vi "Change Speed.vi"(8 "error in (no error)":errorcluster, 10 "Mixer":i16(knob) scale=0.0..100.0, 11 "Feeder Actor.lvlib:Mixer.lvclass":refnum<class "Mixer.lvclass">) -> (0 "error out":errorcluster, 3 "Actor out":refnum<class "Actor.lvclass">)   [LabVIEW 2018, in "Feeder Actor.lvlib" / "Mixer.lvclass"]
uses:
  Mixer.lvclass
  C:/Program Files/National Instruments/LabVIEW 2018/vi.lib/ActorFramework/Actor/Actor.lvclass
  <vilib>/ActorFramework/Actor/Actor.lvclass
  Mixer.lvclass/Mixer.ctl
  <vilib>/DAQmx/write.llb/DAQmx Write (Counter Frequency 1Chan 1Samp).vi
  <vilib>/DAQmx/miscellaneous.llb/DAQmx Fill In Error Info.vi
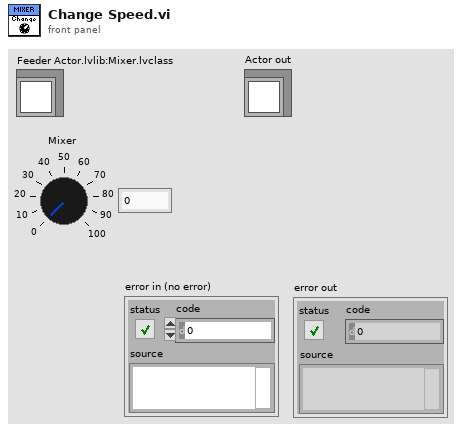
[diagram p1: front panel]
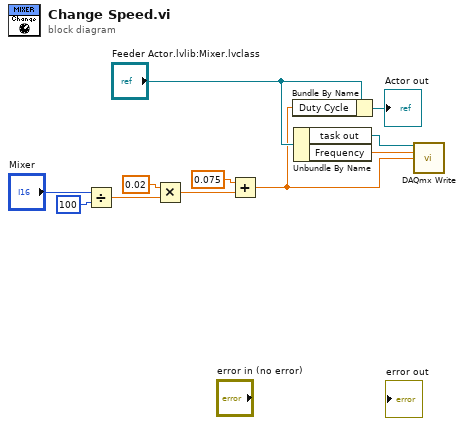
[diagram p0: block diagram]
diagram:
  n1 = Divide(x="Mixer", y=i16 100) -> (x/y=w7:dbl)
  n2 = Multiply(x=0.02, y=w7) -> (x*y=w4:dbl)
  n3 = Add(x=0.075, y=w4) -> (x+y=w2:dbl)
  n4 = Bundle By Name(cluster="Feeder Actor.lvlib:Mixer.lvclass", "Duty Cycle"=w2) -> (→"Actor out":refnum<class "Mixer.lvclass">)
  n5 = Unbundle By Name("Feeder Actor.lvlib:Mixer.lvclass") -> ("task out"=w11:refnum<k21>, "Frequency"=w10:dbl)
  n6 = call-poly <vilib>:"DAQmx Write.vi"("task/channels in"=w11, "frequency"=w10, "duty cycle"=w2) -> ()  [unwired: 10 in, 3 out]
